vi "updateDisplay.vi"(8 "error in (no error)":errorcluster, 11 "PixelflySettings in":refnum<class "PixelflySettings.lvclass">) -> (0 "error out":errorcluster, 3 "PixelflySettings out":refnum<class "PixelflySettings.lvclass">)   [LabVIEW 2009, in "Tools.lvlib" / "Settings.lvlib" / "PixelflySettings.lvclass"]
uses:
  PixelflySettings.lvclass
  PixelflySettings.lvclass/PixelflySettings.ctl
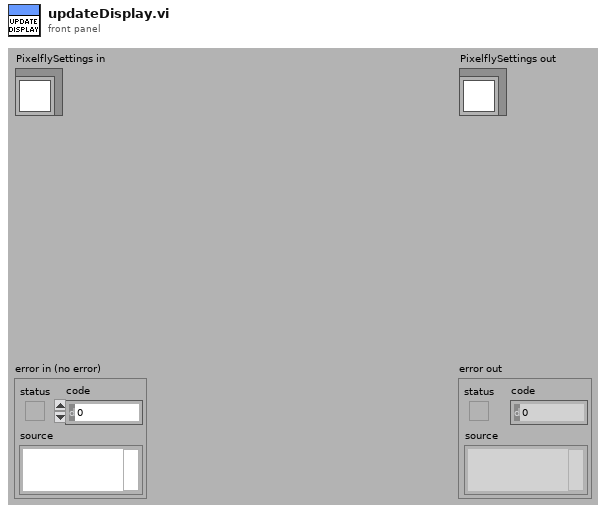
[diagram p1: front panel]
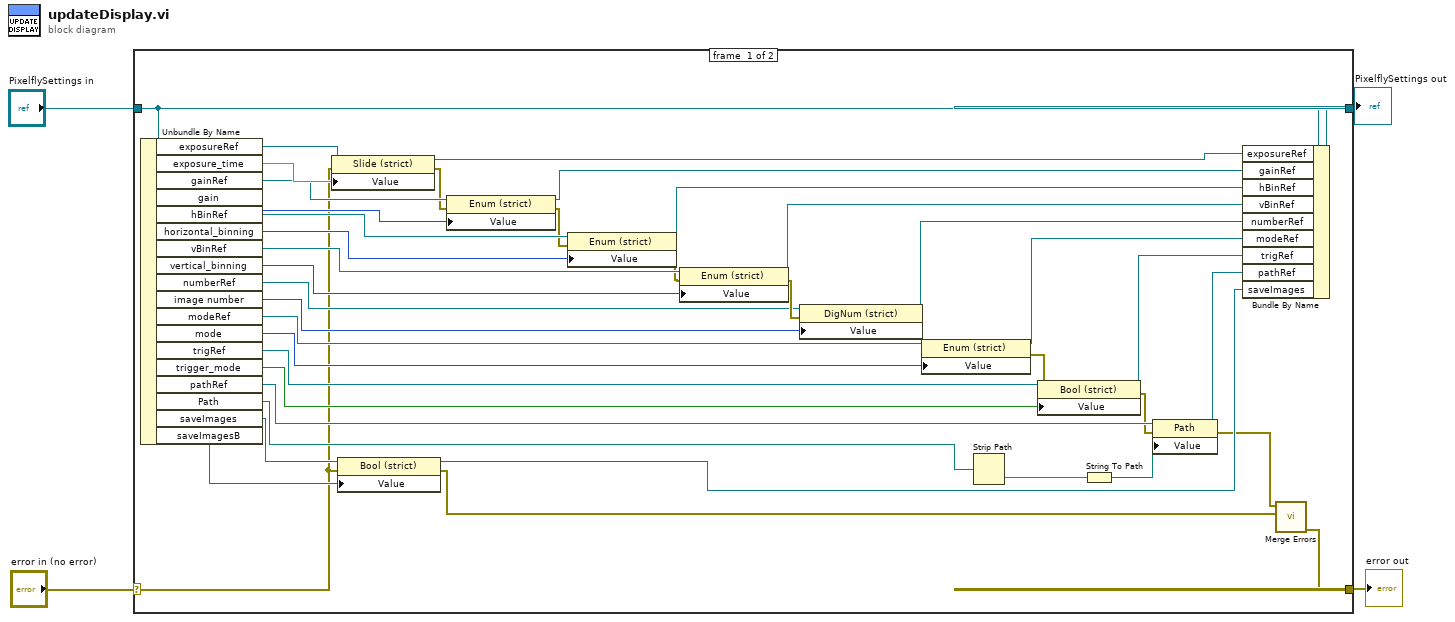
[diagram p0: block diagram]
diagram:
  n1 = case shown="No Error" "error in (no error)" {
    selector: "error in (no error)" -> [w9 w48]
    tunnel: [w5 w48] -> w3
    tunnel: [w18 w47] -> w1
    tunnel: "PixelflySettings in" -> [w19 w47]
    frame #0 {
      n2 = Unbundle By Name(w19) -> ("exposureRef"=w46:refnum<vi>, "exposure_time"=w45:dbl, "gainRef"=w44:refnum<vi>, "gain"=w42:enum16{"Low", "High"}, "hBinRef"=w41:refnum<vi>, "horizontal_binning"=w40:enum16{"1", "2"}, "vBinRef"=w38:refnum<vi>, "vertical_binning"=w36:enum16{"1", "2"}, "numberRef"=w34:refnum<vi>, "image number"=w33:i32, "modeRef"=w32:refnum<vi>, "mode"=w31:u16, "trigRef"=w29:refnum<vi>, "trigger_mode"=w28:bool, "pathRef"=w17:refnum<vi>, "Path"=w14:path, "saveImages"=w11:refnum<vi>, "saveImagesB"=w10:bool)
      n3 = property class="Slide (strict)"(reference=w46, error in=w9, "Value"=w45) -> (reference out=w26:refnum<vi>, error out=w43:errorcluster)
      n4 = property class="Bool (strict)"(reference=w11, error in=w9, "Value"=w10) -> (reference out=w8:refnum<vi>, error out=w6:errorcluster)
      n5 = property class="Enum (strict)"(reference=w44, error in=w43, "Value"=w42) -> (reference out=w25:refnum<vi>, error out=w39:errorcluster)
      n6 = property class="Enum (strict)"(reference=w41, error in=w39, "Value"=w40) -> (reference out=w24:refnum<vi>, error out=w37:errorcluster)
      n7 = property class="Enum (strict)"(reference=w38, error in=w37, "Value"=w36) -> (reference out=w23:refnum<vi>, error out=w35:errorcluster)
      n8 = property class="DigNum (strict)"(reference=w34, error in=w35, "Value"=w33) -> (reference out=w22:refnum<vi>, error out=w30:errorcluster)
      n9 = property class="Enum (strict)"(reference=w32, error in=w30, "Value"=w31) -> (reference out=w21:refnum<vi>, error out=w27:errorcluster)
      n10 = Strip Path(path=w14) -> (name=w13:string)  [unwired: 1 out]
      n11 = property class="Bool (strict)"(reference=w29, error in=w27, "Value"=w28) -> (reference out=w20:refnum<vi>, error out=w16:errorcluster)
      n12 = String To Path(string=w13) -> (path=w12:path)
      n13 = property class="Path"(reference=w17, error in=w16, "Value"=w12) -> (reference out=w15:refnum<vi>, error out=w7:errorcluster)
      n14 = Bundle By Name(cluster=w19, "exposureRef"=w26, "gainRef"=w25, "hBinRef"=w24, "vBinRef"=w23, "numberRef"=w22, "modeRef"=w21, "trigRef"=w20, "pathRef"=w15, "saveImages"=w8) -> (w18:refnum<class "PixelflySettings.lvclass">)
      n15 = call <vilib>:"Merge Errors.vi"("error in 2 (no error)"=w6, "error in 1 (no error)"=w7) -> ("error out"=w5:errorcluster)  [unwired: 5 in]
    }
    frame #1 {
    }
  }
  "error out" <- w3
  "PixelflySettings out" <- w1
